vi "Calc_Actuators_Power Limit Left.vi"(0 "Power IN":dbl, 7 "Elev":dbl, 9 "Elev_Max":dbl, 11 "Elev_Min":dbl) -> (14 "Power OUT":dbl)   [LabVIEW 2017]
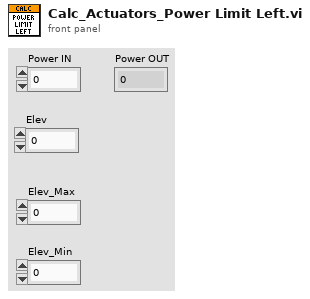
[diagram p1: front panel]
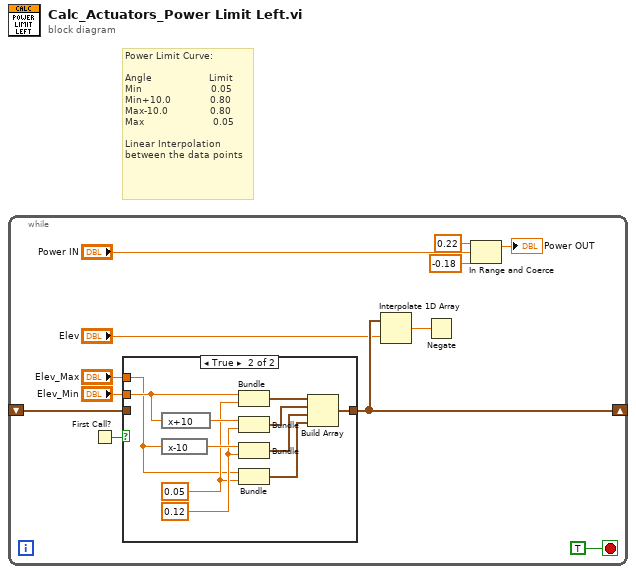
[diagram p0: block diagram]
diagram:
  # "Power Limit Curve:\n\nAngle                   Limit\nMin                       0.05\nMin+10.0             0.80\nMax-10.0              0.80\nMax                       0.05\n\nLinear Interpolation\nbetween the data points"
  n1 = while {
    shift-right: [w8] -> _
    shift-left: _ -> [w9]
    stop <- TRUE stop-if-true
    n2 = First Call?() -> (First Call?: T/F=w12:bool)
    n3 = case shown="True" w12 {
      tunnel: "Elev_Min" -> [_ w24]
      tunnel: "Elev_Max" -> [_ w19]
      tunnel: [w13 w14] -> w8
      tunnel: w9 -> [w13 _]
      frame False {
      }
      frame True {
        w21 = 0.12 ("Limit")
        w20 = 0.05 ("Limit")
        n4 = expression code="x+10"(w24) -> (w23:dbl)
        n5 = expression code="x-10"(w19) -> (w22:dbl)
        n6 = Bundle("Elev_Min"=w24, "Limit"=w20) -> (w18:cluster{"Elev_Min":dbl, "Limit":dbl})  [unwired: 1 in]
        n7 = Bundle("Elev_Min"=w23, "Limit"=w21) -> (w17:cluster{"Elev_Min":dbl, "Limit":dbl})  [unwired: 1 in]
        n8 = Bundle("Elev_Max"=w22, "Limit"=w21) -> (w16:cluster{"Elev_Max":dbl, "Limit":dbl})  [unwired: 1 in]
        n9 = Bundle("Elev_Max"=w19, "Limit"=w20) -> (w15:cluster{"Elev_Max":dbl, "Limit":dbl})  [unwired: 1 in]
        n10 = Build Array(w18, w17, w16, w15) -> (w14:cluster{"Elev_Max":dbl, "Limit":dbl}[])
      }
    }
    n11 = Interpolate 1D Array(1:"Elev", 2:w8) -> (0:w4:dbl)
    n12 = Negate(x=w4) -> ()  [unwired: 1 out]
    n13 = In Range and Coerce(upper limit=0.22, x="Power IN", lower limit=-0.18) -> (coerced(x)=→"Power OUT":dbl)  [unwired: 1 out]
  }
